vi "cota dos espaçadores.vi"(8 "error in":errorcluster, 11 "Dados SP":T1={"Condutor"={"Pc (N/m)"=0.0, "Mod.Young (N/m²)"=0.0, "Dil.Term.c (m/°C)"=0.0, "Área  (m²)"=0.0, "Tração EDS (N)"=0.0, "Tração Torig(N)"=0.0, "Tração Talta (N)"=0.0}, "Suporte"={"Ps (N/m)"=0.0, "Es (N/m²)"=0.0, "DTc (1/°C)"=0.0, "Área sup (m²)"=0.0, "Tração EDS sup (N)"=0.0, "Tração AT sup (N)"=0.0, "Flecha sup AT (m)"=0.0}, "Projeto"={"Temp. EDS (°C)"=0.0, "Lim.original (°C)"=0.0, "Lim.extend. (°C)"=0.0, "N. cabo/fase"=1.0}, "Vetor de dados"={"Coor.X.esp"=[], "Coor.Y.Esp."=[], "Sub.vao X"=[], "Sub.vao Y"=[], "CoordY.sup"=[], "CoordX.sup"=[]}, "Subvão"={"N. Esp."=0.0, "F.lim (m)"=0.0, "Ext.calc"=0.0, "Ext.definido"=0.0, "Comp.cabo"=0.0, "Ext.55%"=0.0, "Tração sub\nAT (N)"=0.0, "Ext.sel."=0.0, "Flecha lim.\ncalc (m)"=0.0}, "Vão"={"Extensão (m)"=0.0, "Desnivel (m)"=0.0, "Ext.Lim sub (m)"=0.0, "Flecha à 60 °C"=0.0}} {"Projeto"."N. cabo/fase" min=1.0 max=8.0 step=1.0 format="%#_1f"}) -> (0 "error out":errorcluster, 3 "Dados SP Out":T1={"Condutor"={"Pc (N/m)"=0.0, "Mod.Young (N/m²)"=0.0, "Dil.Term.c (m/°C)"=0.0, "Área  (m²)"=0.0, "Tração EDS (N)"=0.0, "Tração Torig(N)"=0.0, "Tração Talta (N)"=0.0}, "Suporte"={"Ps (N/m)"=0.0, "Es (N/m²)"=0.0, "DTc (1/°C)"=0.0, "Área sup (m²)"=0.0, "Tração EDS sup (N)"=0.0, "Tração AT sup (N)"=0.0, "Flecha sup AT (m)"=0.0}, "Projeto"={"Temp. EDS (°C)"=0.0, "Lim.original (°C)"=0.0, "Lim.extend. (°C)"=0.0, "N. cabo/fase"=1.0}, "Vetor de dados"={"Coor.X.esp"=[], "Coor.Y.Esp."=[], "Sub.vao X"=[], "Sub.vao Y"=[], "CoordY.sup"=[], "CoordX.sup"=[]}, "Subvão"={"N. Esp."=0.0, "F.lim (m)"=0.0, "Ext.calc"=0.0, "Ext.definido"=0.0, "Comp.cabo"=0.0, "Ext.55%"=0.0, "Tração sub\nAT (N)"=0.0, "Ext.sel."=0.0, "Flecha lim.\ncalc (m)"=0.0}, "Vão"={"Extensão (m)"=0.0, "Desnivel (m)"=0.0, "Ext.Lim sub (m)"=0.0, "Flecha à 60 °C"=0.0}} {"Projeto"."N. cabo/fase" min=1.0 max=8.0 step=1.0 format="%#_1f"})   [LabVIEW 2020]
uses:
  controles/SP data.ctl
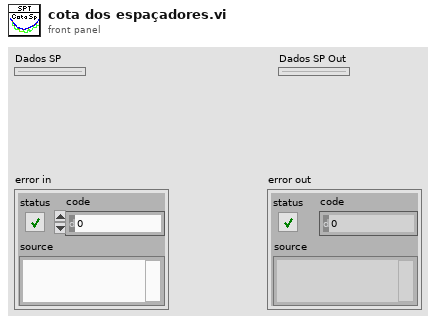
[diagram p1: front panel]
types:
  T1 = typedef "SP data.ctl" = cluster{"Condutor":cluster{"Pc (N/m)":dbl, "Mod.Young (N/m²)":dbl, "Dil.Term.c (m/°C)":dbl, "Área  (m²)":dbl, "Tração EDS (N)":dbl, "Tração Torig(N)":dbl, "Tração Talta (N)":dbl}, "Suporte":cluster{"Ps (N/m)":dbl, "Es (N/m²)":dbl, "DTc (1/°C)":dbl, "Área sup (m²)":dbl, "Tração EDS sup (N)":dbl, "Tração AT sup (N)":dbl, "Flecha sup AT (m)":dbl}, "Projeto":cluster{"Temp. EDS (°C)":dbl, "Lim.original (°C)":dbl, "Lim.extend. (°C)":dbl, "N. cabo/fase":dbl}, "Vetor de dados":cluster{"Coor.X.esp":dbl[], "Coor.Y.Esp.":dbl[], "Sub.vao X":dbl[], "Sub.vao Y":dbl[], "CoordY.sup":dbl[], "CoordX.sup":dbl[]}, "Subvão":cluster{"N. Esp.":dbl, "F.lim (m)":dbl, "Ext.calc":dbl, "Ext.definido":dbl, "Comp.cabo":dbl, "Ext.55%":dbl, "Tração sub\nAT (N)":dbl, "Ext.sel.":dbl, "Flecha lim.\ncalc (m)":dbl}, "Vão":cluster{"Extensão (m)":dbl, "Desnivel (m)":dbl, "Ext.Lim sub (m)":dbl, "Flecha à 60 °C":dbl}}
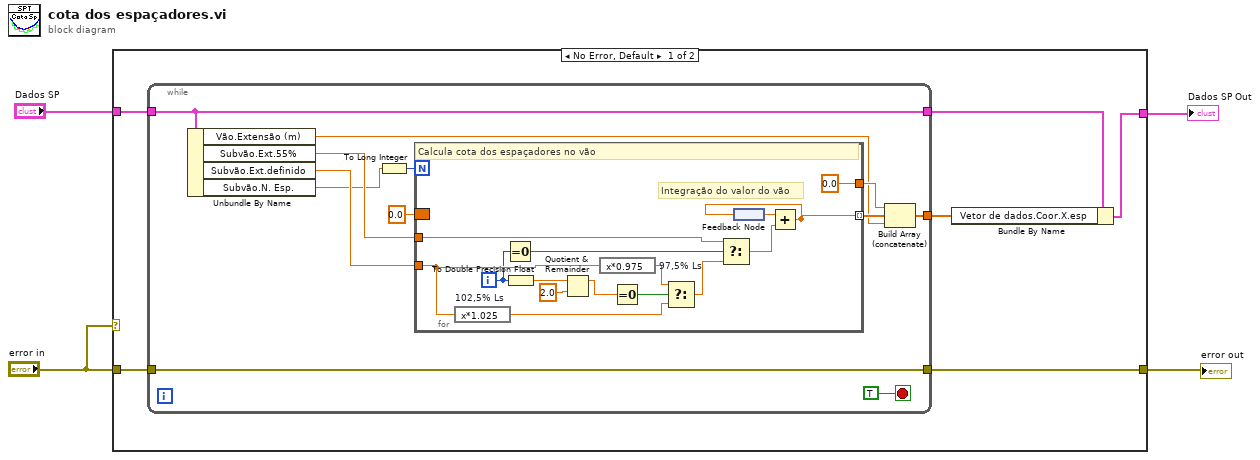
[diagram p0: block diagram]
diagram:
  n1 = case shown="No Error, Default" "error in" {
    tunnel: "Dados SP" -> [w10 w38]
    tunnel: "error in" -> [w9 w39]
    tunnel: [w7 w38] -> w3
    tunnel: [w5 w39] -> w2
    frame No Error {
      n2 = while {
        tunnel: [w21] -> w6
        tunnel: w10 -> [w17]
        tunnel: [w18] -> w5
        tunnel: w9 -> [w18]
        tunnel: [w17] -> w8
        stop <- TRUE stop-if-true
        n3 = Unbundle By Name(w17) -> ("Vão.Extensão (m)"=w19:dbl, "Subvão.Ext.55%"=w15:dbl, "Subvão.Ext.definido"=w14:dbl, "Subvão.N. Esp."=w13:dbl)
        n4 = To Long Integer(number=w13) -> (32bit integer=w12:i32)
        n5 = for {
          N: w12 -> [_]
          tunnel: w14 -> [w33]
          tunnel: w15 -> [w30]
          tunnel: [w25] -> w20 mode=indexing
          tunnel: [0.0] -> w22
          border: 0.0 -> [_]
          i -> [w29]
          # "Integração do valor do vão"
          # "Calcula cota dos espaçadores no vão"
          n6 = expression code="x*1.025" "102,5% Ls"(w33) -> (w32:dbl)
          n7 = Equal To 0?(x=w29) -> (x = 0?=w28:bool)
          n8 = To Double Precision Float(number=w29) -> (double precision float=w24:dbl)
          n9 = Quotient & Remainder(x=w24, y=2.0) -> (x-y*floor(x/y)=w37:dbl)  [unwired: 1 out]
          n10 = expression code="x*0.975" "97,5% Ls"(w33) -> (w35:dbl)
          n11 = Equal To 0?(x=w37) -> (x = 0?=w31:bool)
          n12 = Select(t=w35, s=w31, f=w32) -> (s? t:f=w34:dbl)
          n13 = Select(t=w30, s=w28, f=w34) -> (s? t:f=w27:dbl)
          n14 = feedback #1() -> (w26:dbl)
          n15 = Add(x=w26, y=w27) -> (x+y=w25:dbl)
          n16 = feedback-in #1(w25) -> ()
        }
        n17 = Build Array (concatenate)(w22, w20, w19) -> (w21:dbl[])
      }
      n18 = Bundle By Name(cluster=w8, "Vetor de dados.Coor.X.esp"=w6) -> (w7:T1)
    }
    frame Error {
    }
  }
  "Dados SP Out" <- w3
  "error out" <- w2
